vi "Teleop.vi"(10 "Match Info":T1={"Autonomous Elapsed Seconds"=0.0, "TeleOp Elapsed Seconds"=0.0, "Disabled Elapsed Seconds"=0.0, "Visited Autonomous"=FALSE, "Visited TeleOp"=FALSE, "Visited Disabled"=FALSE, "Autonomous Settings"={"Autonomous Style"=enum."Independent", "VI Refnum"=refnum}}, 11 "Call Context":T2) -> ()   [LabVIEW 2011]
doc: "This VI is called for each TeleOp packet received from the DS where the robot is not disabled. It is often used to read from the joysticks and update I/O or to update setpoints for timed control loops. It should complete and return within 20 milliseconds or it may miss DS packets."
uses:
  <vilib>/Rock Robotics/WPI/DriverStation/WPI_DriverStationDerivedRobotMode.ctl
  <vilib>/Rock Robotics/WPI/DriverStation/WPI_DriverStationMatch Info.ctl
  <vilib>/Rock Robotics/WPI/Relay/WPI_RelayValue.ctl
  Robot Global Data.vi
panel:
  in  "top":bool=TRUE
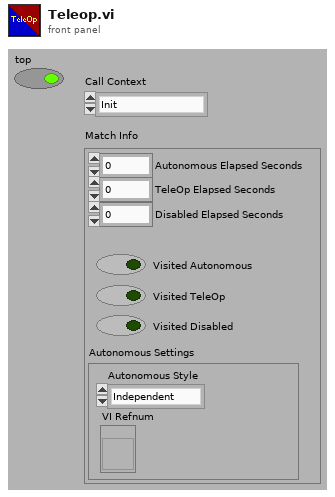
[diagram p1: front panel]
types:
  T1 = typedef "WPI_DriverStationMatch Info.ctl" = cluster{"Autonomous Elapsed Seconds":dbl, "TeleOp Elapsed Seconds":dbl, "Disabled Elapsed Seconds":dbl, "Visited Autonomous":bool, "Visited TeleOp":bool, "Visited Disabled":bool, "Autonomous Settings":cluster{"Autonomous Style":enum16{"Iterative", "Independent"}, "VI Refnum":refnum<vi>}}
  T2 = typedef "WPI_DriverStationDerivedRobotMode.ctl" = enum16{"Init", "Execute", "Stop"}
  T3 = typedef "WPI_DigitalInputDevRef.ctl" = cluster{"DevStatus":errorcluster, "DIO Channel":T4, "Digital Module":T5}
  T4 = typedef "FPGA_DIOChannel.ctl" = enum8{"DIO 1", "DIO 2", "DIO 3", "DIO 4", "DIO 5", "DIO 6", "DIO 7", "DIO 8", "DIO 9", "DIO 10", "DIO 11", "DIO 12", "DIO 13", "DIO 14", "Invalid"}
  T5 = typedef "FPGA_TypedefDigitalModule.ctl" = enum16{"Digital Module 1", "Digital Module 2"}
  T6 = typedef "WPI_GyroDevRef.ctl" = cluster{"DevStatus":errorcluster, "Analog Module":T7, "Analog Channel":T8, "Offset":dbl, "Gain (VoltsPerDegree/Second)":dbl}
  T7 = typedef "FPGA_TypedefAnalogModule.ctl" = enum16{"Analog Module 1", "Analog Module 2"}
  T8 = typedef "FPGA_AIChannel.ctl" = enum8{"AI 1", "AI 2", "AI 3", "AI 4", "AI 5", "AI 6", "AI 7", "AI 8", "Invalid"}
  T9 = typedef "WPI_RobotDriveDevRef.ctl" = cluster{"DevStatus":errorcluster, "Motors[]":T10[], "Square Inputs":bool, "Max Output":dbl, "Isochronous":bool}
  T10 = typedef "WPI_MotorControlDeviceRef.ctl" = cluster{"DeviceStatus":errorcluster, "Type":enum16{"PWM", "CAN"}, "PWM":cluster{"Digital Module":T5, "PWM Channel":T11, "DeadBand":T12}, "CAN":cluster{"Device Number":u8, "Control Mode":T13, "Semaphore":T14, "Max Vout":dbl}, "Invert":bool, "TransformRef":T15, "InvTransformRef":T15}
  T11 = typedef "FPGA_DIOPWMChannel.ctl" = enum8{"PWM 1", "PWM 2", "PWM 3", "PWM 4", "PWM 5", "PWM 6", "PWM 7", "PWM 8", "PWM 9", "PWM 10", "Invalid"}
  T12 = typedef "WPI_PWMDeadband.ctl" = cluster{"Name":string, "maxPositivePwm":i32, "minPositivePwm":i32, "centerPwm":i32, "maxNegativePwm":i32, "minNegativePwm":i32, "angularRange":u16}
  T13 = typedef "WPI_CANJaguar_ControlMode.ctl" = enum8{"Percent VBus", "Current", "Speed", "Position", "Voltage"}
  T14 = typedef "Semaphore RefNum" = refnum<k1>
  T15 = typedef "WPI_PWMTransform_ConPane.ctl" = refnum<vi>
  T16 = typedef "WPI_JoystickDevRef.ctl" = cluster{"Device":T17}
  T17 = typedef "WPI_JoystickDeviceEnum.ctl" = enum16{"USB 1", "USB 2", "USB 3", "USB 4", "Kinect 1", "Kinect 2"}
  T18 = cluster{"Position":cluster{"X":dbl, "Y":dbl}, "Distance (m)":dbl, "Target Found?":bool}
  T19 = typedef "WPI_ServoDeviceRef.ctl" = cluster{"DeviceStatus":errorcluster, "Digital Module":T5, "PWM Channel":T11, "DeadBand":T12}
  T20 = typedef "WPI_EncoderDevRef.ctl" = cluster{"DevStatus":errorcluster, "EncoderIndex":T21, "CounterIndex":T22, "DistancePerCount":dbl, "Decoding Type":T23}
  T21 = typedef "FPGA_EncoderIdx.ctl" = enum8{"Enc 0", "Enc 1", "Enc 2", "Enc 3", "Invalid"}
  T22 = typedef "FPGA_CounterCtrSystemIndex.ctl" = enum8{"Ctr 0", "Ctr 1", "Ctr 2", "Ctr 3", "Ctr 4", "Ctr 5", "Ctr 6", "Ctr 7", "Invalid"}
  T23 = typedef "WPI_EncoderType.ctl" = enum16{"1x", "2x", "4x"}
  T24 = typedef "WPI_RelayValue.ctl" = enum16{"Off", "On", "Forward", "Reverse"}
  T25 = typedef "WPI_RelayDevRef.ctl" = cluster{"DevStatus":errorcluster, "Relay Channel":T26, "Digital Module":T5, "Relay Direction":T27}
  T26 = typedef "FPGA_DIORelayChannel.ctl" = enum8{"Relay 1", "Relay 2", "Relay 3", "Relay 4", "Relay 5", "Relay 6", "Relay 7", "Relay 8", "Invalid"}
  T27 = typedef "WPI_RelayDirection.ctl" = enum16{"Both directions", "Forward only", "Reverse only"}
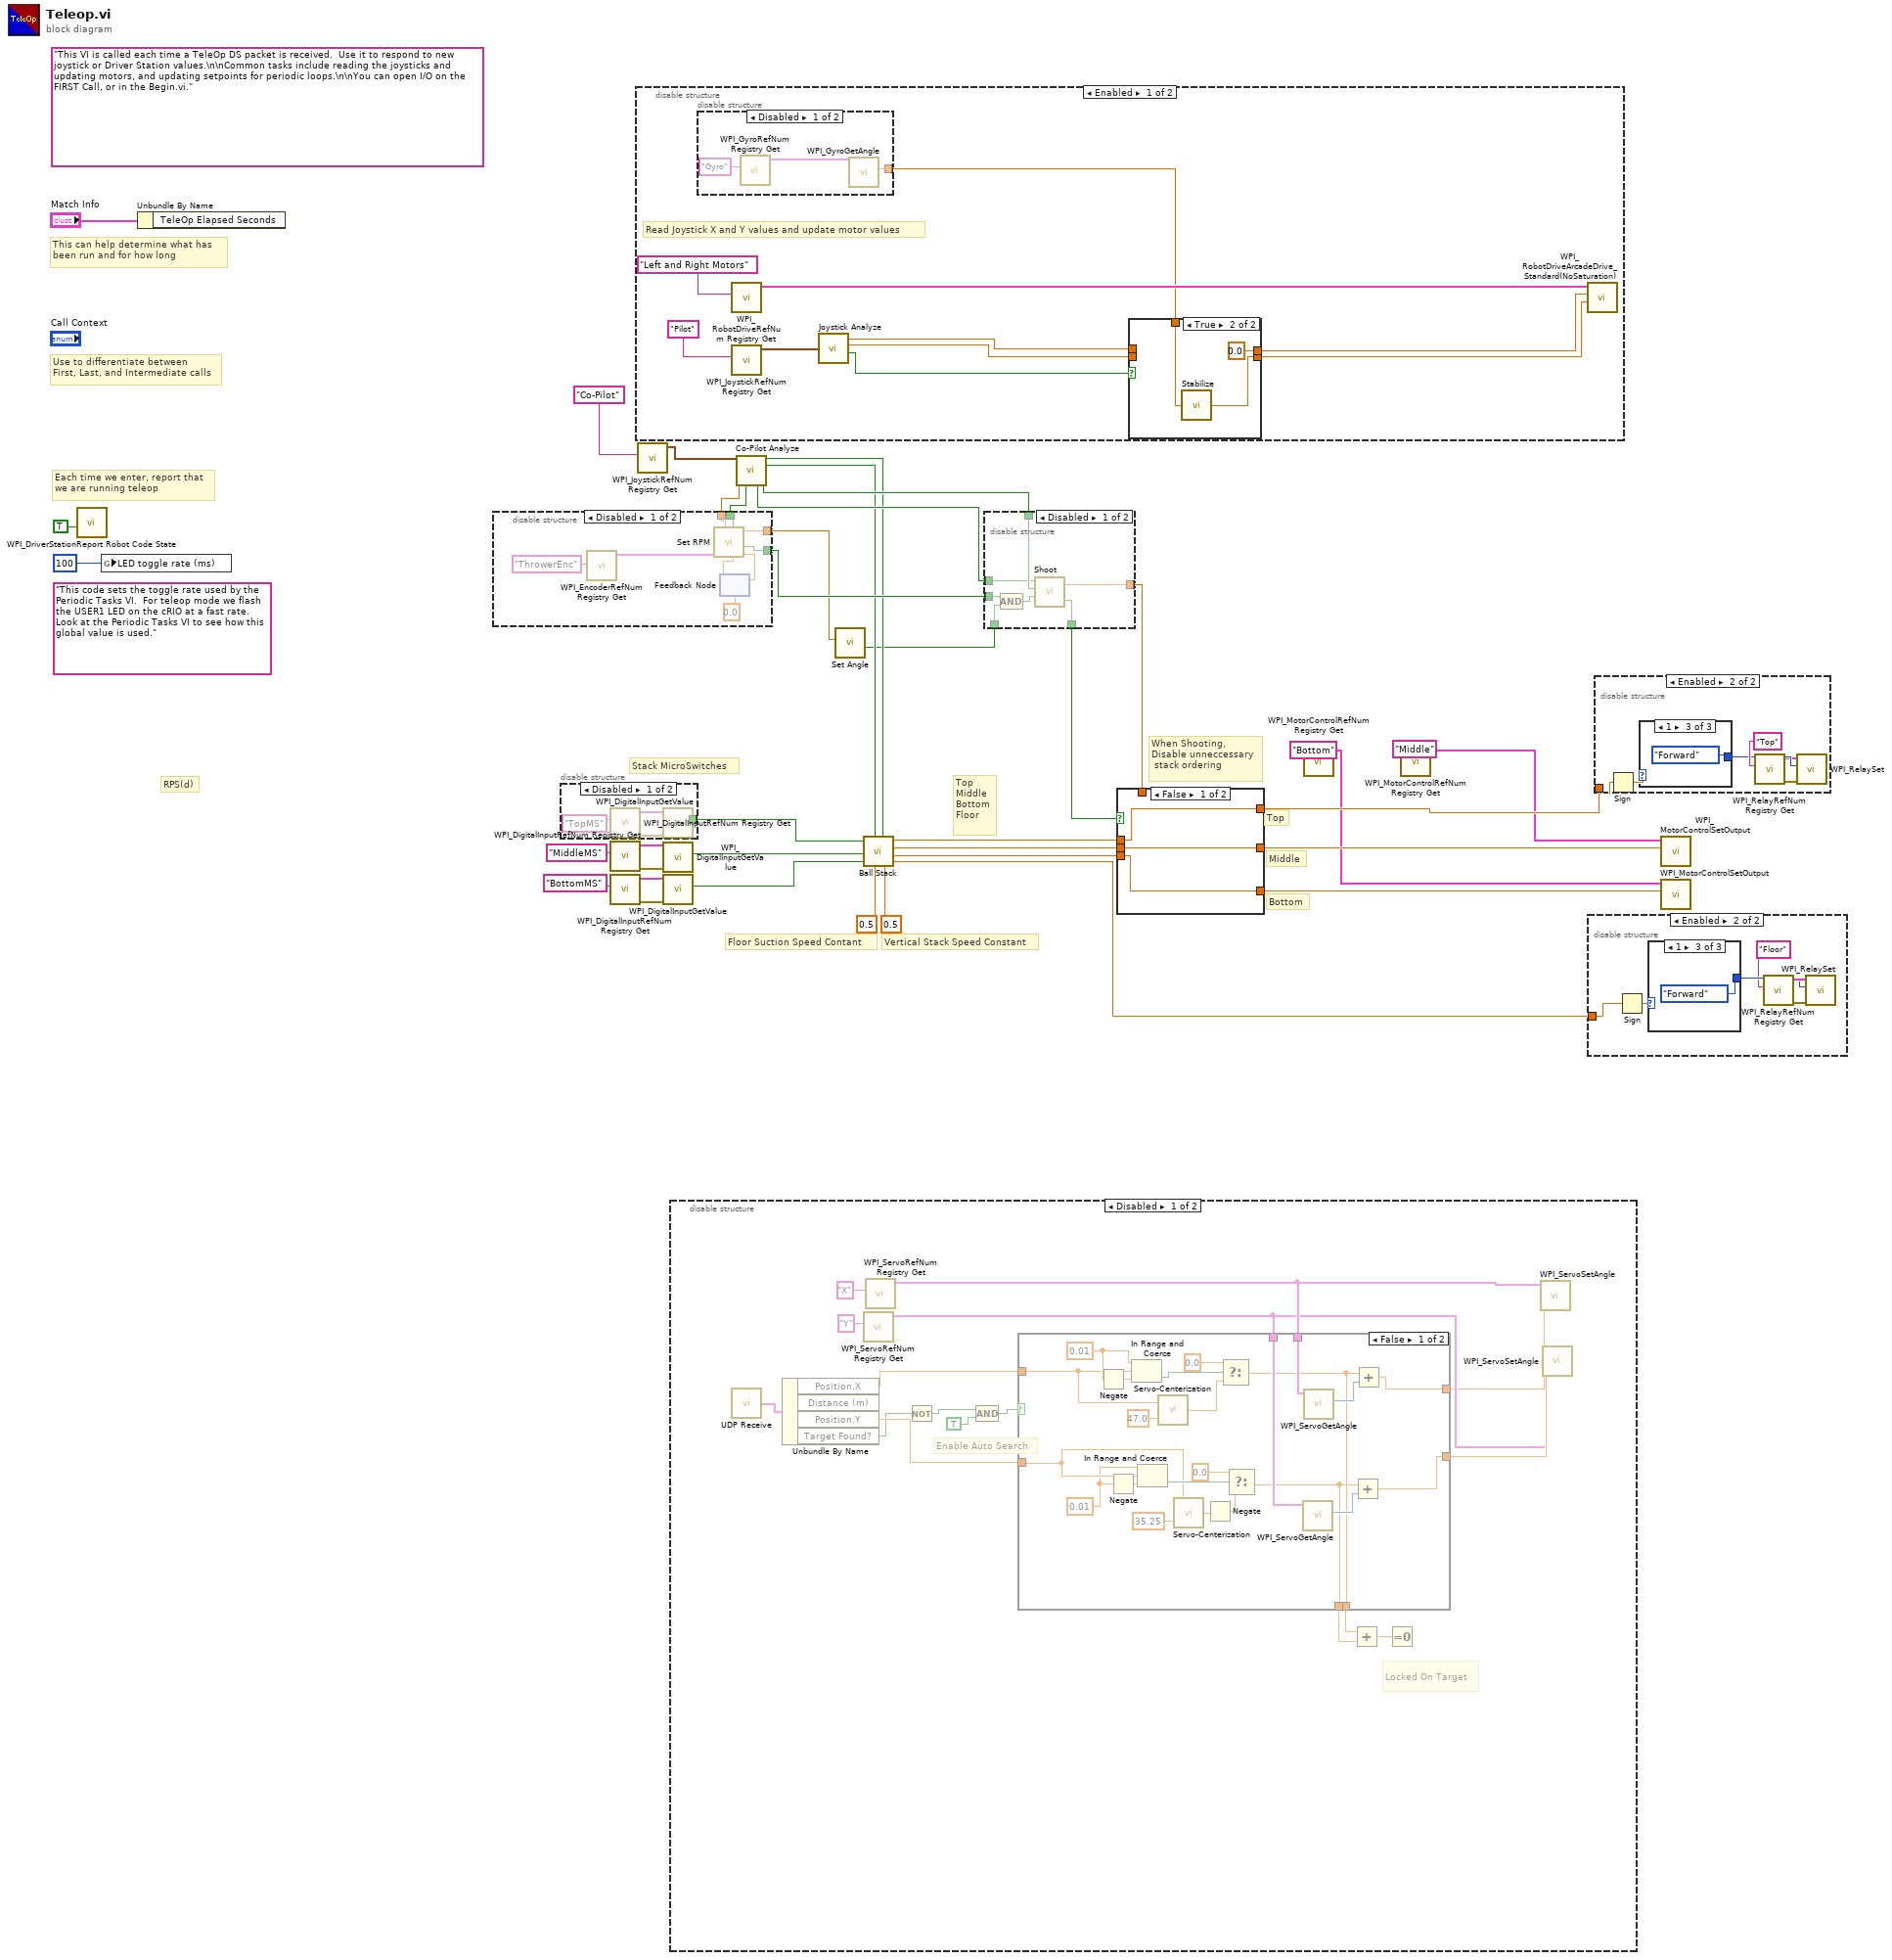
[diagram p0: block diagram]
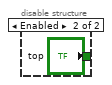
[diagram p2: hidden frame]
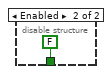
[diagram p7: hidden frame]
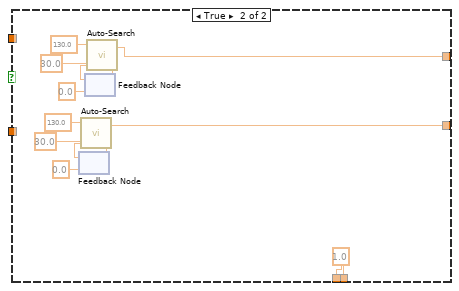
[diagram p8: hidden frame]
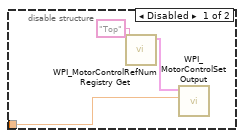
[diagram p10: hidden frame]
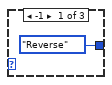
[diagram p11: hidden frame]
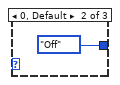
[diagram p12: hidden frame]
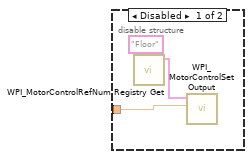
[diagram p13: hidden frame]
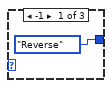
[diagram p14: hidden frame]
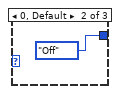
[diagram p15: hidden frame]
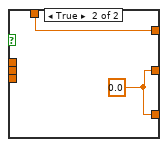
[diagram p16: hidden frame]
diagram:
  (unwired) "This code sets the toggle rate used by the Periodic Tasks VI.  For teleop mode we flash the USER1 LED on the cRIO at a fast rate.  Look at the Periodic Tasks VI to see how this global value is used."
  (unwired) "This VI is called each time a TeleOp DS packet is received.  Use it to respond to new joystick or Driver Station values.\n\nCommon tasks include reading the joysticks and updating motors, and updating setpoints for periodic loops.\n\nYou can open I/O on the FIRST Call, or in the Begin.vi."
  # "RPS(d)"
  # "Stack MicroSwitches"
  # "Top\nMiddle\nBottom\nFloor"
  # "Floor Suction Speed Contant"
  # "Vertical Stack Speed Constant"
  # "When Shooting,\nDisable unneccessary\n stack ordering"
  # "Bottom"
  # "Middle"
  # "Top"
  # "Each time we enter, report that\nwe are running teleop"
  # "Use to differentiate between\nFirst, Last, and Intermediate calls"
  # "This can help determine what has\nbeen run and for how long"
  n1 = call <vilib>:"WPI_DriverStationReport Robot Code State.vi"("TeleOp"=TRUE ("Autonomous")) -> ()  [unwired: 10 in, 1 out]
  n2 = global write "Robot Global Data.vi" "LED toggle rate (ms)"(u32 100 ("LED ms toggle rate")) -> ()
  n3 = Unbundle By Name("Match Info") -> ()  [unwired: 1 out]
  n4 = disable-structure shown="Disabled" {
    disable-tunnel: [w39 "top"] -> w13
    frame Disabled {
      n5 = call <vilib>:"WPI_DigitalInputRefNum Registry Get.vi"("refnum name"="TopMS") -> ("error out"=w41:errorcluster, "DigitalInputDevRef"=w40:T3)  [unwired: 9 in]
      n6 = call <vilib>:"WPI_DigitalInputGetValue.vi"("error in (no error)"=w41, "DigitalInputDevRef"=w40) -> ("Value"=w39:bool)  [unwired: 7 in, 2 out]
    }
    frame Enabled {
    }
  }
  n7 = call <vilib>:"WPI_DigitalInputRefNum Registry Get.vi"("refnum name"="MiddleMS") -> ("error out"=w17:errorcluster, "DigitalInputDevRef"=w16:T3)  [unwired: 9 in]
  n8 = call <vilib>:"WPI_DigitalInputRefNum Registry Get.vi"("refnum name"="BottomMS") -> ("error out"=w15:errorcluster, "DigitalInputDevRef"=w14:T3)  [unwired: 9 in]
  n9 = disable-structure shown="Enabled" {
    frame Enabled {
      # "Read Joystick X and Y values and update motor values"
      n10 = disable-structure shown="Disabled" {
        disable-tunnel: [w54 _] -> w44
        frame Disabled {
          n11 = call <vilib>:"WPI_GyroRefNum Registry Get.vi"("refnum name"="Gyro") -> ("GyroDevRef"=w55:T6)  [unwired: 9 in, 1 out]
          n12 = call <vilib>:"WPI_GyroGetAngle.vi"("GyroDevRef"=w55) -> ("Angle"=w54:dbl)  [unwired: 7 in, 3 out]
        }
        frame Enabled {
        }
      }
      n13 = call <vilib>:"WPI_RobotDriveRefNum Registry Get.vi"("refnum name"="Left and Right Motors") -> ("RobotDriveDevRef"=w52:T9)  [unwired: 1 in, 9 out]
      n14 = call <vilib>:"WPI_JoystickRefNum Registry Get.vi"("refnum name"="Pilot") -> ("JoystickDevRef"=w50:T16)  [unwired: 1 in, 9 out]
      n15 = call "Joystick Analyze.vi"("Joystick Name"=w50) -> ("x"=w47:dbl, "y"=w48:dbl, "Stabilize"=w45:bool)  [unwired: 7 in]
      n16 = case shown="True" w45 {
        tunnel: [w58 w60] -> w49
        tunnel: w48 -> [w58 _]
        tunnel: [w57 0.0 ("x")] -> w46
        tunnel: w47 -> [w57 _]
        tunnel: w44 -> [_ w59]
        frame False {
        }
        frame True {
          n17 = call "Stabilize.vi"("Angle"=w59) -> ("result"=w60:dbl)
        }
      }
      n18 = call <vilib>:"WPI_RobotDriveArcadeDrive_Standard(NoSaturation).vi"("Y axis value"=w49, "X axis value"=w46, "RobotDriveDevRef"=w52) -> ()  [unwired: 1 in, 8 out]
    }
    frame Disabled {
    }
  }
  n19 = call <vilib>:"WPI_JoystickRefNum Registry Get.vi"("refnum name"="Co-Pilot") -> ("JoystickDevRef"=w9:T16)  [unwired: 1 in, 9 out]
  n20 = call <vilib>:"WPI_DigitalInputGetValue.vi"("error in (no error)"=w17, "DigitalInputDevRef"=w16) -> ("Value"=w12:bool)  [unwired: 7 in, 2 out]
  n21 = call <vilib>:"WPI_DigitalInputGetValue.vi"("error in (no error)"=w15, "DigitalInputDevRef"=w14) -> ("Value"=w11:bool)  [unwired: 7 in, 2 out]
  n22 = disable-structure shown="Disabled" {
    frame Disabled {
      # "Locked On Target"
      # "Enable Auto Search"
      n23 = call "UDP Receive.vi"() -> ("Selected Target Info"=w77:T18)  [unwired: 1 in]
      n24 = Unbundle By Name(w77) -> ("Position.X"=w73:dbl, "Position.Y"=w72:dbl, "Target Found?"=w63:bool)  [unwired: 1 out]
      n25 = call <vilib>:"WPI_ServoRefNum Registry Get.vi"("refnum name"="Y") -> ("ServoDeviceRef"=w70:T19)  [unwired: 9 in, 1 out]
      n26 = call <vilib>:"WPI_ServoRefNum Registry Get.vi"("refnum name"="X") -> ("ServoDeviceRef"=w71:T19)  [unwired: 9 in, 1 out]
      n27 = Not(x=w63) -> (.not. x?=w62:bool)
      n28 = Compound Arithmetic op=AND(w62, TRUE ("y")) -> (w64:bool)
      n29 = case shown="False" w64 {
        tunnel: [w83 w108] -> w69
        tunnel: [w82 w102] -> w74
        tunnel: w72 -> [w91 _]
        tunnel: w73 -> [w88 _]
        tunnel: w71 -> [w81 _]
        tunnel: w70 -> [w80 _]
        tunnel: [w79 w101] -> w68
        tunnel: [w78 w101] -> w67
        frame False {
          w87 = 0.01 ("lower limit")
          w89 = 0.01 ("upper limit")
          n30 = Negate(x=w89) -> (-x=w90:dbl)
          n31 = Negate(x=w87) -> (-x=w86:dbl)
          n32 = In Range and Coerce(upper limit=w89, x=w88, lower limit=w90) -> (In Range?=w92:bool)  [unwired: 1 out]
          n33 = In Range and Coerce(upper limit=w87, x=w91, lower limit=w86) -> (In Range?=w93:bool)  [unwired: 1 out]
          n34 = call "Servo-Centerization.vi"("Camera Angle"=47.0 ("HALF Cam angle constant"), "Cartez"=w88) -> ("Rounded Error"=w95:dbl)
          n35 = call "Servo-Centerization.vi"("Camera Angle"=35.25 ("HALF Cam angle constant"), "Cartez"=w91) -> ("Rounded Error"=w99:dbl)
          n36 = Negate(x=w99) -> (-x=w100:dbl)
          n37 = Select(t=0.0 ("f"), s=w92, f=w95) -> (s? t:f=w79:dbl)
          n38 = Select(t=0.0 ("f"), s=w93, f=w100) -> (s? t:f=w78:dbl)
          n39 = call <vilib>:"WPI_ServoGetAngle.vi"("ServoDeviceRef"=w80) -> ("Angle"=w85:u16)  [unwired: 7 in, 2 out]
          n40 = call <vilib>:"WPI_ServoGetAngle.vi"("ServoDeviceRef"=w81) -> ("Angle"=w84:u16)  [unwired: 7 in, 2 out]
          n41 = Add(x=w78, y=w85) -> (x+y=w82:dbl)
          n42 = Add(x=w79, y=w84) -> (x+y=w83:dbl)
        }
        frame True {
          w101 = 1.0 ("Rounded Error")
          n43 = feedback #1(0.0 ("counter")) -> (w106:dbl)
          n44 = call "Auto-Search.vi"("Counter\\Timer"=w106, "Low Angle Edge"=30.0, "High Angle Edge"=130.0) -> ("counter"=w105:dbl, "Servo Angle"=w102:dbl)
          n45 = feedback-in #1(w105) -> ()
          n46 = feedback #2(0.0 ("counter")) -> (w110:dbl)
          n47 = call "Auto-Search.vi"("Counter\\Timer"=w110, "Low Angle Edge"=30.0, "High Angle Edge"=130.0) -> ("counter"=w111:dbl, "Servo Angle"=w108:dbl)
          n48 = feedback-in #2(w111) -> ()
        }
      }
      n49 = Add(x=w68, y=w67) -> (x+y=w66:dbl)
      n50 = Equal To 0?(x=w66) -> ()  [unwired: 1 out]
      n51 = call <vilib>:"WPI_ServoSetAngle.vi"("Angle"=w69, "ServoDeviceRef"=w71) -> ()  [unwired: 8 in, 2 out]
      n52 = call <vilib>:"WPI_ServoSetAngle.vi"("Angle"=w74, "ServoDeviceRef"=w70) -> ()  [unwired: 8 in, 2 out]
    }
    frame Enabled {
    }
  }
  n53 = call "Co-Pilot Analyze.vi"("JoystickDevRef"=w9) -> ("Suction"=w5:bool, "Ejection"=w6:bool, "Fine Tune(RPM)"=w4:dbl, "Fine Tune?"=w3:bool, "Fire Override"=w7:bool, "Fire"=w8:bool)  [unwired: 9 in]
  n54 = disable-structure shown="Disabled" {
    disable-tunnel: [w122 _] -> w35
    disable-tunnel: w4 -> [w119 _]
    disable-tunnel: w3 -> [w118 _]
    disable-tunnel: [w114 _] -> w1
    frame Disabled {
      n55 = call <vilib>:"WPI_EncoderRefNum Registry Get.vi"("refnum name"="ThrowerEnc") -> ("EncoderDevRef"=w121:T20)  [unwired: 9 in, 1 out]
      n56 = feedback #3(0.0 ("Thrower Voltage")) -> (w116:dbl)
      n57 = call "Set RPM.vi"("Last Thrower Voltage (node)"=w116, "Fine Tune?"=w118, "Fine Tuning"=w119, "EncoderDevRef"=w121) -> ("Thrower Voltage"=w117:dbl, "RPM SET"=w122:bool, "angle"=w114:dbl)  [unwired: 5 in]
      n58 = feedback-in #3(w117) -> ()
    }
    frame Enabled {
    }
  }
  n59 = call "Set Angle.vi"("Angle"=w1) -> ("Angle SET"=w2:bool)  [unwired: 9 in, 1 out]
  n60 = call "Ball Stack.vi"("top"=w13, "spinOut"=w6, "middle"=w12, "bottom"=w11, "suckMotorSpeed"=0.5, "suck"=w5, "Vertical Stack Speed"=0.5) -> ("topMotor"=w20:dbl, "middleMotor"=w21:dbl, "bottomMotor"=w22:dbl, "suckMotor"=w23:dbl)
  n61 = disable-structure shown="Disabled" {
    disable-tunnel: w35 -> [w125 _]
    disable-tunnel: [w129 FALSE ("Le Fire at Will?")] -> w34
    disable-tunnel: [w128 _] -> w33
    disable-tunnel: w8 -> [w127 _]
    disable-tunnel: w7 -> [w126 _]
    disable-tunnel: w2 -> [w123 _]
    frame Disabled {
      n62 = Compound Arithmetic op=AND(w125, w123) -> (w124:bool)
      n63 = call "Shoot.vi"("Ready 2 Shoot?"=w124, "Fire"=w127, "Override"=w126) -> ("Le Fire at Will?"=w129:bool, "Top"=w128:dbl)  [unwired: 1 in]
    }
    frame Enabled {
    }
  }
  n64 = case shown="False" w34 {
    tunnel: [w133 w135] -> w32
    tunnel: w33 -> [_ w135]
    tunnel: [w132 w134] -> w31
    tunnel: [w131 w134] -> w30
    tunnel: w22 -> [w131 _]
    tunnel: w21 -> [w132 _]
    tunnel: w20 -> [w133 _]
    frame False {
    }
    frame True {
      w134 = 0.0 ("Top")
    }
  }
  n65 = call <vilib>:"WPI_MotorControlRefNum Registry Get.vi"("refnum name"="Bottom") -> ("MotorControlDevRef"=w28:T10)  [unwired: 9 in, 1 out]
  n66 = call <vilib>:"WPI_MotorControlRefNum Registry Get.vi"("refnum name"="Middle") -> ("MotorControlDevRef"=w29:T10)  [unwired: 9 in, 1 out]
  n67 = disable-structure shown="Enabled" {
    disable-tunnel: w23 -> [w136 w139]
    frame Disabled {
      n68 = call <vilib>:"WPI_MotorControlRefNum Registry Get.vi"("refnum name"="Floor") -> ("MotorControlDevRef"=w137:T10)  [unwired: 9 in, 1 out]
      n69 = call <vilib>:"WPI_MotorControlSetOutput.vi"("Output"=w136, "MotorControlDevRef"=w137) -> ()  [unwired: 8 in, 2 out]
    }
    frame Enabled {
      n70 = Sign(1:w139) -> (0:w144:dbl)
      n71 = case shown="1" w144 {
        tunnel: [WPI_RelayValue."Reverse" ("RelayValue") WPI_RelayValue."Off" ("RelayValue") WPI_RelayValue."Forward" ("RelayValue")] -> w141
        frame -1 {
        }
        frame 0, Default {
        }
        frame 1 {
        }
      }
      n72 = call <vilib>:"WPI_RelayRefNum Registry Get.vi"("refnum name"="Floor") -> ("error out"=w143:errorcluster, "RelayDevRef"=w142:T25)  [unwired: 9 in]
      n73 = call <vilib>:"WPI_RelaySet.vi"("error in (no error)"=w143, "RelayValue"=w141, "RelayDevRef"=w142) -> ()  [unwired: 7 in, 2 out]
    }
  }
  n74 = disable-structure shown="Enabled" {
    disable-tunnel: w32 -> [w150 w151]
    frame Disabled {
      n75 = call <vilib>:"WPI_MotorControlRefNum Registry Get.vi"("refnum name"="Top") -> ("MotorControlDevRef"=w149:T10)  [unwired: 9 in, 1 out]
      n76 = call <vilib>:"WPI_MotorControlSetOutput.vi"("Output"=w150, "MotorControlDevRef"=w149) -> ()  [unwired: 8 in, 2 out]
    }
    frame Enabled {
      n77 = Sign(1:w151) -> (0:w152:dbl)
      n78 = case shown="1" w152 {
        tunnel: [WPI_RelayValue."Reverse" ("RelayValue") WPI_RelayValue."Off" ("RelayValue") WPI_RelayValue."Forward" ("RelayValue")] -> w155
        frame -1 {
        }
        frame 0, Default {
        }
        frame 1 {
        }
      }
      n79 = call <vilib>:"WPI_RelayRefNum Registry Get.vi"("refnum name"="Top") -> ("error out"=w153:errorcluster, "RelayDevRef"=w154:T25)  [unwired: 9 in]
      n80 = call <vilib>:"WPI_RelaySet.vi"("error in (no error)"=w153, "RelayValue"=w155, "RelayDevRef"=w154) -> ()  [unwired: 7 in, 2 out]
    }
  }
  n81 = call <vilib>:"WPI_MotorControlSetOutput.vi"("Output"=w31, "MotorControlDevRef"=w29) -> ()  [unwired: 8 in, 2 out]
  n82 = call <vilib>:"WPI_MotorControlSetOutput.vi"("Output"=w30, "MotorControlDevRef"=w28) -> ()  [unwired: 8 in, 2 out]
